vi "Abort.vi"(8 "error in (no error)":errorcluster, 11 "Bar in":refnum<class "Bar.lvclass">) -> (0 "error out":errorcluster, 3 "Bar out":refnum<class "Bar.lvclass">)   [LabVIEW 2015, in "Simple Progress Bar.lvlib" / "Bar.lvclass"]
doc: "Inform the progress bar user interface that the process has been aborted in order to disable cancel button and enable done button."
uses:
  Bar.lvclass
  Bar.lvclass/Bar.ctl
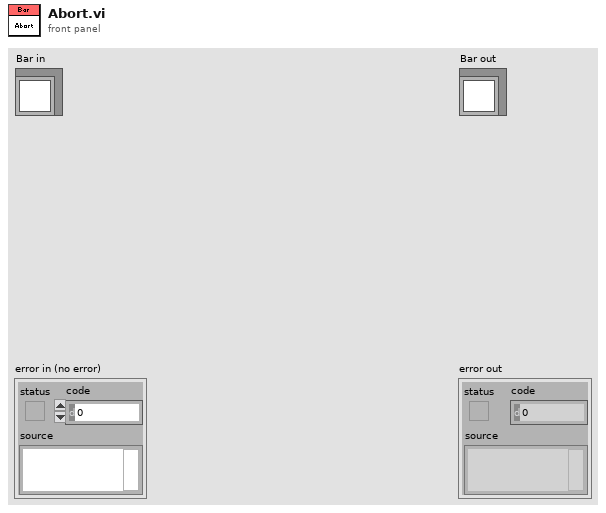
[diagram p1: front panel]
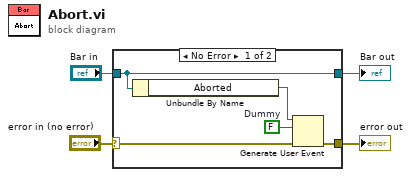
[diagram p0: block diagram]
diagram:
  n1 = case shown="No Error" "error in (no error)" {
    selector: "error in (no error)" -> [w6 w11]
    tunnel: [w5 w11] -> w3
    tunnel: [w7 w10] -> w1
    tunnel: "Bar in" -> [w7 w10]
    frame No Error {
      w8 = FALSE  # Dummy
      n2 = Unbundle By Name(w7) -> ("Aborted"=w9:refnum<user-event>)
      n3 = Generate User Event(user event=w9, event data cluster=w8, error in=w6) -> (error out=w5:errorcluster)  [unwired: 1 in, 1 out]
    }
    frame Error {
    }
  }
  "error out" <- w3
  "Bar out" <- w1
